vi "ExampleMeasurementServer.vi"() -> ()   [LabVIEW 2019]
uses:
  Labview-lrms-proof-of-concept/Tesla-LRMS-PoC/JSONDefaults.ctl
  VIs/labview-grpc-measurement-server.lvlib
  VIs/MeasurementServer_ErrorOutData.ctl
panel:
  in  "Server Key File (.key)":path
  in  "Server Certificate File (.crt)":path
  in  "stop":bool
  in  "Server Address":string="0.0.0.0:50051"
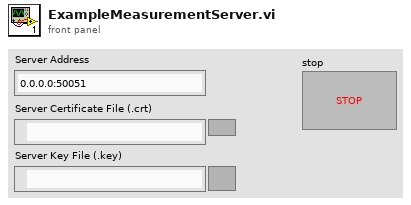
[diagram p1: front panel]
types:
  T1 = typedef "labview-grpc-measurement-server.lvlib/MeasurementServer_gRPCid.ctl" = u64
  T2 = cluster{"QueryServer_Invoke":refnum<user-event>, "QueryServer_Query":refnum<user-event>, "QueryServer_Register":refnum<user-event>, "QueryServer_FourProbeMeasurement":refnum<user-event>, "QueryServer_StreamFourProbeMeasurement":refnum<user-event>, "QueryServer_SendConfig":refnum<user-event>, "QueryServer_StreamError":refnum<user-event>, "gRPCid":T1}
  T3 = typedef "labview-grpc-measurement-server.lvlib/MeasurementServer_ErrorOutData.ctl" = cluster{"ErrorCode":i32, "ErrorMessage":string}
  T4 = typedef "JSONDefaults.ctl" = string[]
  T5 = typedef "labview-grpc-measurement-server.lvlib/MeasurementServer_FourProbeRawData.ctl" = cluster{"Positive Voltage":dbl, "Positive Current":dbl, "Negative Voltage":dbl, "Negative Current":dbl, "Impedance":dbl, "ErrorOutData":T3}
  T6 = typedef "labview-grpc-measurement-server.lvlib/MeasurementServer_ConfigRequest.ctl" = cluster{"SMUResourceName":string, "SMUChannels":string, "SMUSourceMode":i32, "SMUOutputFunction":i32, "SMUSourceTransientResponse":i32, "SMUCurrent":sgl, "SMUCurrentLevelRange":sgl, "SMUMeasurementSense":i32, "SMUMeasurementApertureTime":sgl, "SMUSourceAdvancedSourceDelay":sgl, "SMUVoltage":sgl, "SMUSourceAdvancedSequenceLoopCount":i32, "SMUMeasurementAdvancedDCNoiseRejection":i32, "SMUSequenceName":string, "ScanList":string, "DMMResourceName":string, "DMMFunction":i32, "DMMResolution":sgl, "DMMRange":sgl, "DMMSampleCount":i32, "DMMApertureTimeUnit":i32, "DMMApertureTime":sgl, "DMMNumberOfAverages":i32, "DMMAutoZero":i32, "DMMADCCalibration":i32, "DMMSettleTime":sgl, "DMMControlAction":i32, "DMMVoltageFaultUpperLimit":sgl, "ApplicationNumberOfWeldChannels":i32}
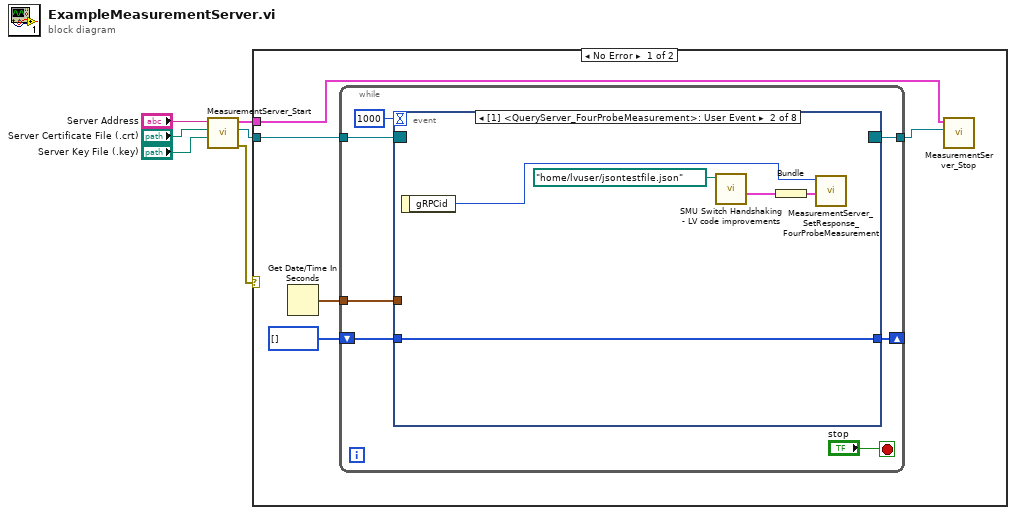
[diagram p0: block diagram]
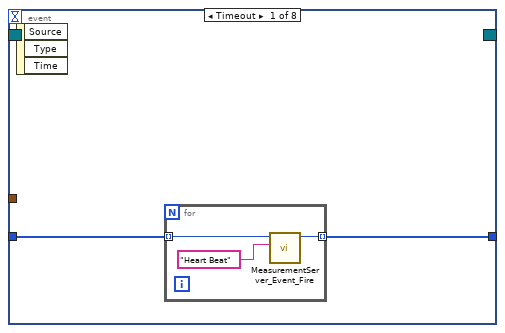
[diagram p2: hidden frame]
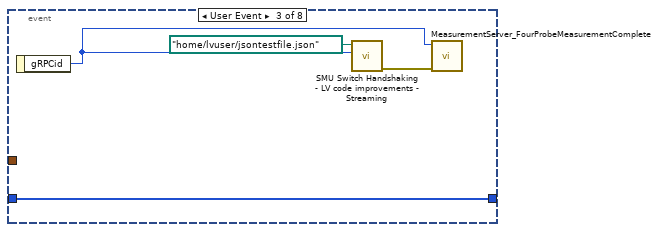
[diagram p3: hidden frame]
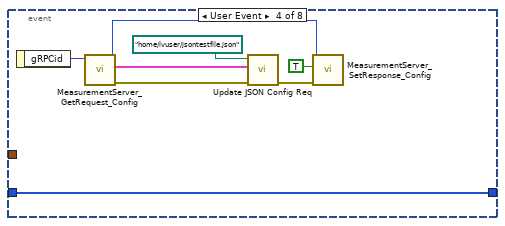
[diagram p4: hidden frame]
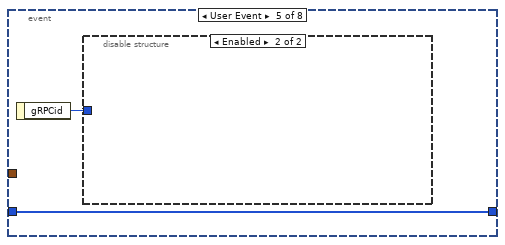
[diagram p5: hidden frame]
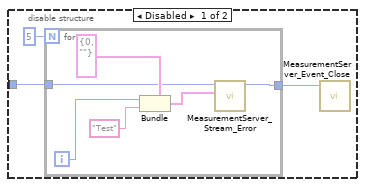
[diagram p6: hidden frame]
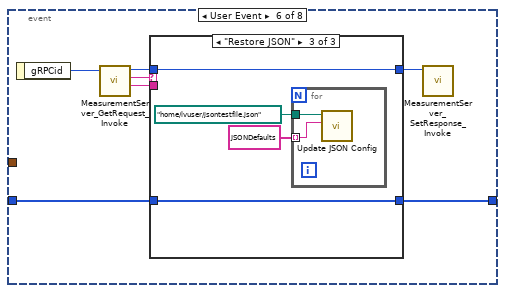
[diagram p7: hidden frame]
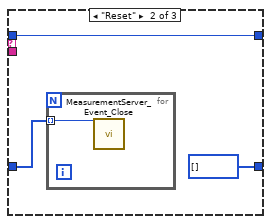
[diagram p9: hidden frame]
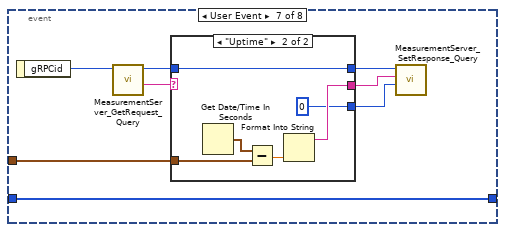
[diagram p10: hidden frame]
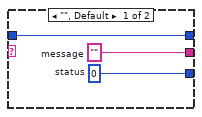
[diagram p11: hidden frame]
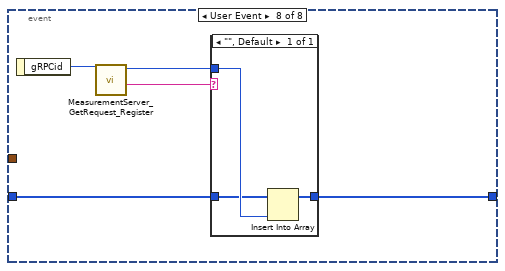
[diagram p12: hidden frame]
diagram:
  n1 = call "MeasurementServer_Start.vi"("Server Key File (.key)"="Server Key File (.key)", "Server Certificate File (.crt)"="Server Certificate File (.crt)", "Server Address"="Server Address") -> ("error out"=w2:errorcluster, "Event Registration Refnum"=w1:refnum<event-registration>, "Server Information"=w5:T2)  [unwired: 5 in]
  n2 = case shown="No Error" w2 {
    tunnel: w5 -> [w9 _]
    tunnel: w1 -> [w8 _]
    frame No Error {
      n3 = Get Date/Time In Seconds() -> (seconds since 1Jan1904=w11:timestamp)
      n4 = while {
        tunnel: [w17] -> w7
        tunnel: w11 -> [w16]
        shift-right: [w14] -> _
        shift-left: u64[] [] -> [w13]
        tunnel: w8 -> [w12]
        stop <- "stop" stop-if-true
        n5 = event shown="[1] <QueryServer_FourProbeMeasurement>: User Event" {
          selector: w12 -> [_ _ _ _ _ _ _ _]
          dyn-events: [_ _ _ _ _ _ _ _] -> w17
          timeout: 1000 -> [_ _ _ _ _ _ _ _]
          tunnel: w16 -> [_ _ _ _ _ _ w73 _]
          tunnel: [w20 w28 w32 w37 w41 w52 w72 w90] -> w14
          tunnel: w13 -> [w19 w28 w32 w37 w41 w53 w72 w89]
          event Timeout {
            n6 = event-data() -> ()  [unwired: 1 in, 3 out]
            n7 = for {
              tunnel: w19 -> [w23] mode=indexing
              tunnel: [w21] -> w20 mode=indexing
              n8 = call "MeasurementServer_Event_Fire.vi"("eventdata"="Heart Beat", "gRPCid"=w23) -> ("gRPCid out"=w21:T1)  [unwired: 8 in, 1 out]
            }
          }
          event User Event {
            n9 = event-data() -> ("gRPCid"=w24:T1)  [unwired: 1 in]
            n10 = call "SMU Switch Handshaking - LV code improvements.vi"("file path (use dialog)"=path "/home/lvuser/jsontestfile.json") -> ("Results"=w26:T5[])  [unwired: 8 in, 2 out]
            n11 = Bundle("Results"=w26) -> (w27:cluster{"Results":T5[]})  [unwired: 1 in]
            n12 = call "MeasurementServer_SetResponse_FourProbeMeasurement.vi"("gRPCid"=w24, "FourProbeResponse"=w27) -> ()  [unwired: 8 in, 1 out]
          }
          event User Event {
            n13 = event-data() -> ("gRPCid"=w29:T1)  [unwired: 1 in]
            n14 = call "SMU Switch Handshaking - LV code improvements - Streaming.vi"("gRPCid"=w29, "file path (use dialog)"=path "/home/lvuser/jsontestfile.json") -> ("error out"=w31:errorcluster)  [unwired: 8 in, 1 out]
            n15 = call "MeasurementServer_FourProbeMeasurementComplete.vi"("gRPCid"=w29, "error in (no error)"=w31) -> ()  [unwired: 8 in, 1 out]
          }
          event User Event {
            n16 = event-data() -> ("gRPCid"=w40:T1)  [unwired: 1 in]
            n17 = call "MeasurementServer_GetRequest_Config.vi"("gRPCid"=w40) -> ("error out"=w34:errorcluster, "ConfigRequest"=w35:T6, "gRPCid out"=w39:T1)  [unwired: 6 in]
            n18 = call "Update JSON Config Req.vi"("error in (no error)"=w34, "ConfigRequest"=w35, "JSON Configuration File (.json)"=path "/home/lvuser/jsontestfile.json") -> ("error out"=w33:errorcluster)  [unwired: 8 in]
            n19 = call "MeasurementServer_SetResponse_Config.vi"("gRPCid"=w39, "acknowledge"=TRUE, "error in (no error)"=w33) -> ()  [unwired: 7 in, 1 out]
          }
          event User Event {
            n20 = event-data() -> ("gRPCid"=w42:T1)  [unwired: 1 in]
            n21 = disable-structure shown="Enabled" {
              disable-tunnel: w42 -> [w43 _]
              frame Disabled {
                n22 = for {
                  N: 5 -> [_]
                  tunnel: [w47] -> w44
                  tunnel: w43 -> [w48]
                  i -> [w50]
                  n23 = Bundle(cluster=T3 {"ErrorCode"=0, "ErrorMessage"=""} ("ErrorOutData"), "ErrorCode"=w50, "ErrorMessage"="Test") -> (w46:T3)
                  n24 = call "MeasurementServer_Stream_Error.vi"("ErrorOutData"=w46, "gRPCid"=w48) -> ("gRPCid out"=w47:T1)  [unwired: 8 in, 1 out]
                }
                n25 = call "MeasurementServer_Event_Close.vi"("gRPCid"=w44) -> ()  [unwired: 9 in, 1 out]
              }
              frame Enabled {
              }
            }
          }
          event User Event {
            n26 = event-data() -> ("gRPCid"=w58:T1)  [unwired: 1 in]
            n27 = call "MeasurementServer_GetRequest_Invoke.vi"("gRPCid"=w58) -> ("parameter"=w54:string, "command"=w57:string, "gRPCid out"=w56:T1)  [unwired: 5 in, 1 out]
            n28 = case shown="\"Restore JSON\"" w57 {
              tunnel: w56 -> [w60 w61 w68]
              tunnel: [w60 w61 w68] -> w55
              tunnel: w54 -> [_ _ _]
              tunnel: w53 -> [w59 w63 w67]
              tunnel: [w59 u64[] [] w67] -> w52
              frame "", Default {
              }
              frame "Reset" {
                n29 = for {
                  tunnel: w63 -> [w64] mode=indexing
                  n30 = call "MeasurementServer_Event_Close.vi"("gRPCid"=w64) -> ()  [unwired: 9 in, 1 out]
                }
              }
              frame "Restore JSON" {
                n31 = for {
                  tunnel: path "/home/lvuser/jsontestfile.json" ("JSON Configuration File (.json)") -> [w69]
                  tunnel: T4 ["SETCONF=SMUResourceName[[CONFPARAM]]=SMU", "SETCONF=SMUChannels[[CONFPARAM]]=0", "SETCONF=SMUSourceMode[[CONFPARAM]]=1021", "SETCONF=SMUOutputFunction[[CONFPARAM]]=1007", "SETCONF=SMUSourceTransientResponse[[CONFPARAM]]=1039", "SETCONF=SMUCurrent[[CONFPARAM]]=1.0", "SETCONF=SMUCurrentLevelRange[[CONFPARAM]]=1.0", "SETCONF=SMUMeasurementSense[[CONFPARAM]]=1008", "SETCONF=SMUMeasurementApertureTime[[CONFPARAM]]=0.010", "SETCONF=SMUSourceAdvancedSourceDelay[[CONFPARAM]]=0.000100", "SETCONF=SMUVoltage[[CONFPARAM]]=6", "SETCONF=SMUSourceAdvancedSequenceLoopCount[[CONFPARAM]]=571", "SETCONF=SMUMeasurementAdvancedDCNoiseRejection[[CONFPARAM]]=1044", "SETCONF=SMUSequenceName[[CONFPARAM]]=MySequence", "SETCONF=SMUStep1_Source_DCCurrent_CurrentLevel[[CONFPARAM]]=1150009", "SETCONF=SMUStep2_Measurement_ApertureTime[[CONFPARAM]]=1150058", "SETCONF=SMUStep3_Source_Advanced_SourceDelay[[CONFPARAM]]=1150051", "SETCONF=SMUSequenceNumberOfSteps[[CONFPARAM]]=3", "SETCONF=Switch1ResourceName[[CONFPARAM]]=2526_1", "SETCONF=Switch1Topology[[CONFPARAM]]=2526/2-Wire 79x1 Mux", "SETCONF=Switch1ScanList[[CONFPARAM]]=ch70:75->com", "SETCONF=Switch2ResourceName[[CONFPARAM]]=SwitchBlock1Dev1", "SETCONF=Switch2Topology[[CONFPARAM]]=Configured Topology", "SETCONF=Switch2ScanList[[CONFPARAM]]=[c2->card1r2->c26], [c3->card1r3->c27]; [c6->card1r2->c26], [c7->card1r3->c27]; [c10->card1r2->c26], [c11->card1r3->c27]; [c14->card1r2->c26], [c15->card1r3->c27]; [c18->card1r2->c26], [c19->card1r3->c27]; [c22->card1r2->c26], [c23->card1r3->c27];", "SETCONF=DMMResourceName[[CONFPARAM]]=DMM", "SETCONF=DMMFunction[[CONFPARAM]]=0", "SETCONF=DMMResolution[[CONFPARAM]]=0.1", "SETCONF=DMMRange[[CONFPARAM]]=0.1", "SETCONF=DMMSampleCount[[CONFPARAM]]=0", "SETCONF=DMMApertureTimeUnit[[CONFPARAM]]=0", "SETCONF=DMMApertureTime[[CONFPARAM]]=0.010", "SETCONF=DMMNumberOfAverages[[CONFPARAM]]=1", "SETCONF=DMMAutoZero[[CONFPARAM]]=0", "SETCONF=DMMADCCalibration[[CONFPARAM]]=0", "SETCONF=DMMSettleTime[[CONFPARAM]]=0.0001", "SETCONF=DMMControlAction[[CONFPARAM]]=0", "SETCONF=DMMVoltageFaultUpperLimit[[CONFPARAM]]=0.000050", "SETCONF=ApplicationNumberOfWeldChannels[[CONFPARAM]]=6"] ("JSON Defaults") -> [w70] mode=indexing
                  n32 = call "Update JSON Config.vi"("Parameter and Value"=w70, "JSON Configuration File (.json)"=w69) -> ()  [unwired: 9 in, 1 out]
                }
              }
            }
            n33 = call "MeasurementServer_SetResponse_Invoke.vi"("gRPCid"=w55) -> ()  [unwired: 9 in, 1 out]
          }
          event User Event {
            n34 = event-data() -> ("gRPCid"=w78:T1)  [unwired: 1 in]
            n35 = call "MeasurementServer_GetRequest_Query.vi"("gRPCid"=w78) -> ("gRPCid out"=w77:T1, "query"=w71:string)  [unwired: 7 in, 1 out]
            n36 = case shown="\"Uptime\"" w71 {
              tunnel: w77 -> [w81 w83]
              tunnel: [w81 w83] -> w76
              tunnel: [w80 w84] -> w75
              tunnel: [w79 0 ("status")] -> w74
              tunnel: w73 -> [_ w86]
              frame "", Default {
                w79 = 0  # status
                w80 = ""  # message
              }
              frame "Uptime" {
                n37 = Get Date/Time In Seconds() -> (seconds since 1Jan1904=w87:timestamp)
                n38 = Subtract(x=w87, y=w86) -> (x-y=w85:dbl)
                n39 = Format Into String(w85) -> (resulting string=w84:string)  [unwired: 3 in, 1 out]
              }
            }
            n40 = call "MeasurementServer_SetResponse_Query.vi"("gRPCid"=w76, "message"=w75, "status"=w74) -> ()  [unwired: 7 in, 1 out]
          }
          event User Event {
            n41 = event-data() -> ("gRPCid"=w92:T1)  [unwired: 1 in]
            n42 = call "MeasurementServer_GetRequest_Register.vi"("gRPCid"=w92) -> ("gRPCid out"=w91:T1, "eventname"=w88:string)  [unwired: 7 in, 1 out]
            n43 = case shown="\"\", Default" w88 {
              tunnel: w91 -> [w95]
              tunnel: [w94] -> w90
              tunnel: w89 -> [w93]
              frame "", Default {
                n44 = Insert Into Array(array=w93, new element=w95) -> (w94:T1[])  [unwired: 1 in]
              }
            }
          }
        }
      }
      n45 = call "MeasurementServer_Stop.vi"("Server Information"=w9, "Event Registration Refnum"=w7) -> ()  [unwired: 8 in, 1 out]
    }
    frame Error {
    }
  }
